vi "Helmholtz2D_FEM_Triangulation_Init.vi"(9 "# of unknown":i32, 10 "Y In":dbl[](array[numeric]), 11 "X In":dbl[](array[numeric])) -> (0 "Triangulation":i32[][](array[numeric]), 1 "Edges":i32[][](array[numeric]), 2 "Y Out":dbl[](array[numeric]), 3 "X Out":dbl[](array[numeric]))   [LabVIEW 2017, in "NI_PDE.lvlib"]
uses:
  <vilib>/gmath/NI_PDE.lvlib
  <vilib>/Analysis/1siggen.llb/Ramp Pattern by Samples.vi
  <vilib>/Analysis/NI_AALBase.lvlib
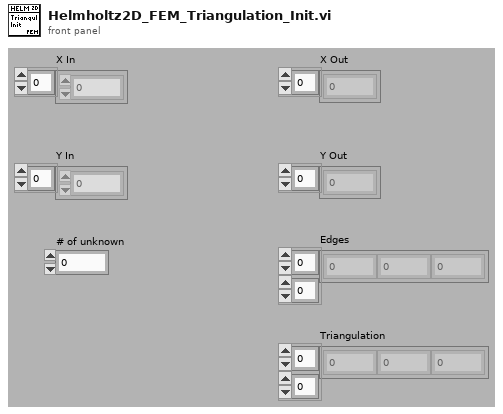
[diagram p1: front panel]
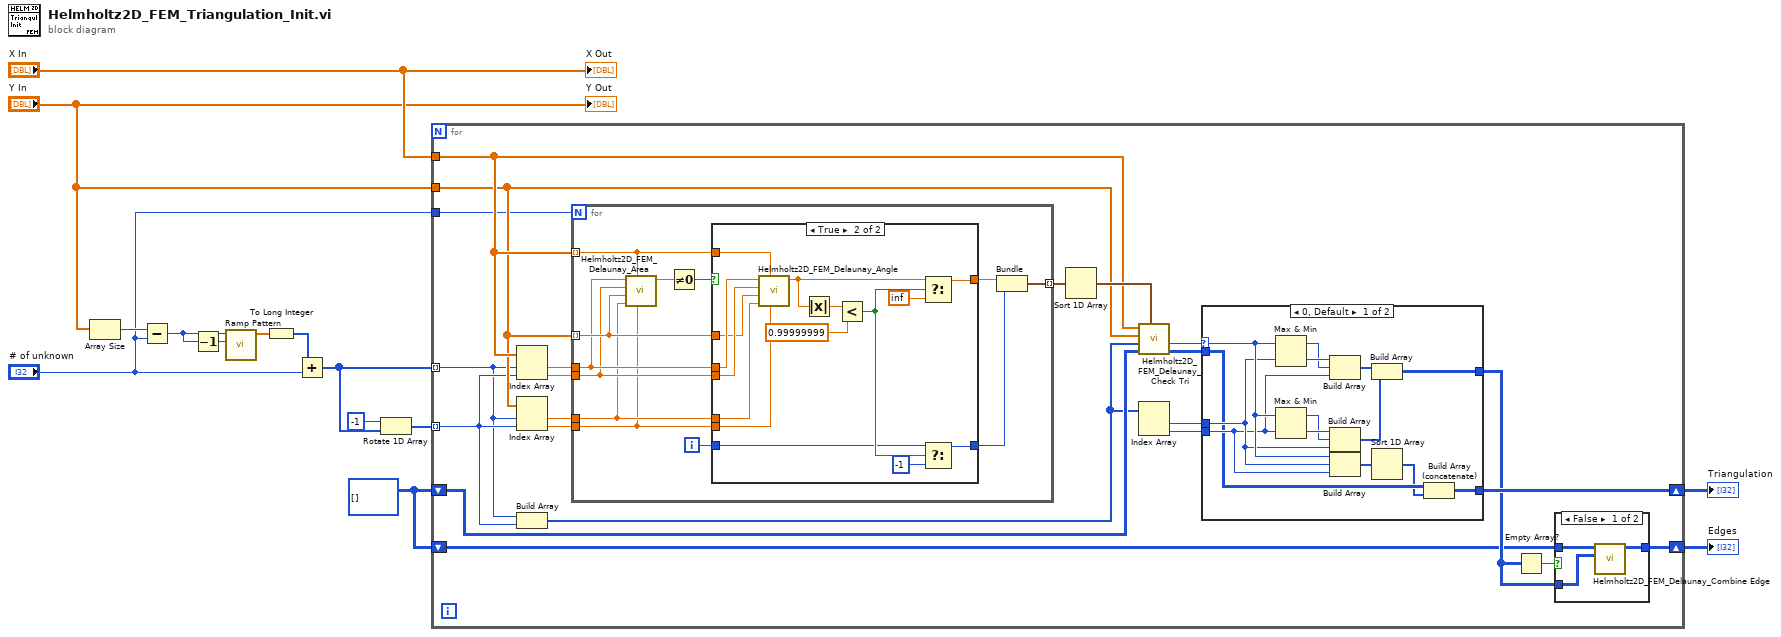
[diagram p0: block diagram]
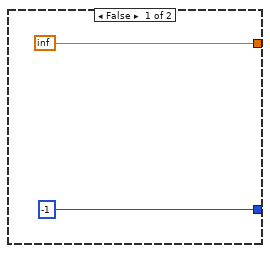
[diagram p4: hidden frame]
diagram:
  w3 = i32[][] [] ("Triangles Out")
  n1 = Array Size(array="Y In") -> (size(s)=w12:i32)
  n2 = Subtract(x=w12, y="# of unknown") -> (x-y=w11:i32)
  n3 = Decrement(x=w11) -> (x-1=w10:i32)
  n4 = call-poly <vilib>:"Ramp Pattern.vi"("end"=w10, "samples"=w11) -> ("Ramp Pattern"=w9:dbl[])  [unwired: 8 in, 1 out]
  n5 = To Long Integer(number=w9) -> (32bit integer=w6:i32[])
  n6 = Add(x=w6, y="# of unknown") -> (x+y=w5:i32[])
  n7 = Rotate 1D Array(1:w5, 2:-1 ("n")) -> (0:w8:i32[])
  n8 = for {
    tunnel: "X In" -> [w25]
    tunnel: "Y In" -> [w24]
    tunnel: "# of unknown" -> [w23]
    shift-right: [w22] -> w13
    shift-left: w3 -> [w30]
    tunnel: w5 -> [w15] mode=indexing
    tunnel: w8 -> [w20] mode=indexing
    shift-right: [w18] -> w14
    shift-left: w3 -> [w16]
    n9 = Index Array(array=w25, index #1=w15, index #2=w20) -> (element #1=w36:dbl, element #2=w35:dbl)
    n10 = Index Array(array=w24, index #1=w15, index #2=w20) -> (element #1=w34:dbl, element #2=w33:dbl)
    n11 = Build Array(w15, w20) -> (w21:i32[])
    n12 = for {
      N: w23 -> [_]
      tunnel: w25 -> [w66] mode=indexing
      tunnel: w24 -> [w65] mode=indexing
      tunnel: w36 -> [w64]
      tunnel: w35 -> [w63]
      tunnel: w34 -> [w62]
      tunnel: w33 -> [w61]
      tunnel: [w57] -> w32 mode=indexing
      i -> [w67]
      n13 = call <vilib>:"Helmholtz2D_FEM_Delaunay_Area.vi"("y3"=w61, "x1"=w66, "y2"=w62, "y1"=w65, "x3"=w63, "x2"=w64) -> ("area"=w60:dbl)  [unwired: 5 out]
      n14 = Not Equal To 0?(x=w60) -> (x != 0?=w56:bool)
      n15 = case shown="True" w56 {
        tunnel: w67 -> [_ w72]
        tunnel: w66 -> [_ w84]
        tunnel: w65 -> [_ w81]
        tunnel: w64 -> [_ w83]
        tunnel: w63 -> [_ w82]
        tunnel: w62 -> [_ w80]
        tunnel: w61 -> [_ w79]
        tunnel: [inf w74] -> w59
        tunnel: [-1 ("y") w71] -> w58
        frame False {
        }
        frame True {
          n16 = call <vilib>:"Helmholtz2D_FEM_Delaunay_Angle.vi"("y3"=w79, "x1"=w84, "y2"=w80, "y1"=w81, "x3"=w82, "x2"=w83) -> ("angle"=w75:dbl)  [unwired: 5 out]
          n17 = Absolute Value(x=w75) -> (abs(x)=w78:dbl)
          n18 = Less?(x=w78, y=0.99999999) -> (x < y?=w73:bool)
          n19 = Select(t=w75, s=w73, f=inf) -> (s? t:f=w74:dbl)
          n20 = Select(t=w72, s=w73, f=-1) -> (s? t:f=w71:i32)
        }
      }
      n21 = Bundle("angle"=w59, "f"=w58) -> (w57:cluster{"angle":dbl, "f":i32})  [unwired: 1 out]
    }
    n22 = Sort 1D Array(array=w32) -> (sorted array=w31:cluster{"angle":dbl, "f":i32}[])
    n23 = call <vilib>:"Helmholtz2D_FEM_Delaunay_Check Tri.vi"("Angle"=w31, "Triangles In"=w30, "Index"=w21, "Y"=w24, "X"=w25) -> ("Triangles Out"=w26:i32[][], "new index"=w29:i32)  [unwired: 5 out]
    n24 = Index Array(array=w21) -> (element #1=w28:i32, element #2=w27:i32)  [unwired: 2 in]
    n25 = case shown="0, Default" w29 {
      selector: w29 -> [w47 _]
      tunnel: w27 -> [w45 _]
      tunnel: w28 -> [w46 _]
      tunnel: [w48 _] -> w17
      tunnel: w26 -> [w43 w55]
      tunnel: [w41 w55] -> w22
      frame 0, Default {
        n26 = Max & Min(x=w47, y=w46) -> (max(x,y)=w53:i32, min(x,y)=w54:i32)
        n27 = Max & Min(x=w47, y=w45) -> (max(x,y)=w51:i32, min(x,y)=w52:i32)
        n28 = Build Array(w54, w53, w45) -> (w50:i32[])
        n29 = Build Array(w52, w51, w46) -> (w49:i32[])
        n30 = Build Array(w47, w46, w45) -> (w44:i32[])
        n31 = Build Array(w50, w49) -> (w48:i32[][])
        n32 = Sort 1D Array(array=w44) -> (sorted array=w42:i32[])
        n33 = Build Array (concatenate)(w43, w42) -> (w41:i32[][])
      }
      frame ..-1 {
      }
    }
    n34 = Empty Array?(array=w17) -> (empty?=w19:bool)
    n35 = case shown="False" w19 {
      tunnel: w16 -> [w39 w40]
      tunnel: [w38 w40] -> w18
      tunnel: w17 -> [w37 _]
      frame False {
        n36 = call <vilib>:"Helmholtz2D_FEM_Delaunay_Combine Edge.vi"("New Edges"=w37, "Edges in"=w39) -> ("Edges Out"=w38:i32[][])  [unwired: 9 out]
      }
      frame True {
      }
    }
  }
  "Triangulation" <- w13
  "Edges" <- w14
  "X Out" <- "X In"
  "Y Out" <- "Y In"
